vi "SubVI_ShifterControl.vi"(2 "Joystick Button":bool, 3 "Number of milliseconds\nto fire solenoids for":i32=200, 4 "Number of milliseconds to wait between shifts.\n~20ms precision.":i32=250) -> (0 "Low Gear Solenoid":bool=TRUE, 1 "High Gear Solenoid":bool=TRUE)   [LabVIEW 2017]
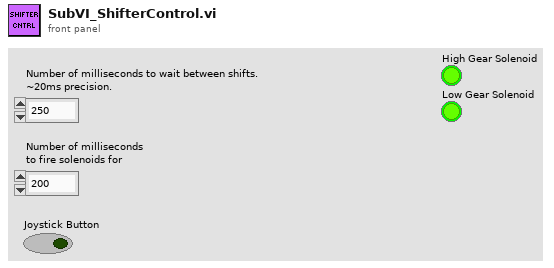
[diagram p1: front panel]
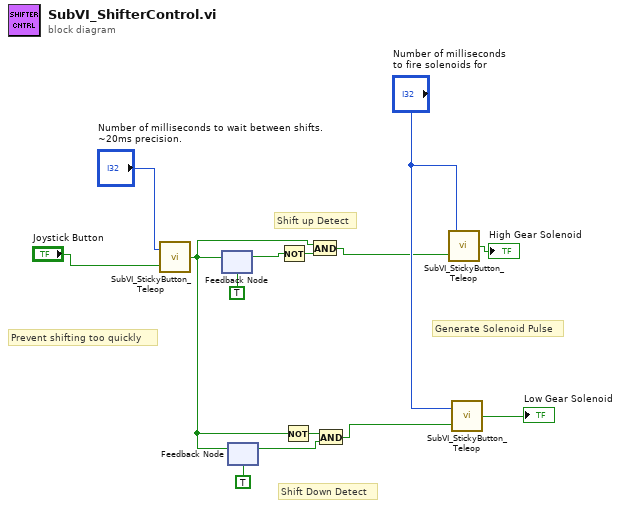
[diagram p0: block diagram]
diagram:
  # "Prevent shifting too quickly"
  # "Generate Solenoid Pulse"
  # "Shift Down Detect"
  # "Shift up Detect"
  n1 = call "SubVI_StickyButton_Teleop.vi"("Speedy Input"="Joystick Button", "Number of milliseconds to wait.\n~20ms precision."="Number of milliseconds to wait between shifts.\n~20ms precision.") -> ("Sticky Output"=w1:bool)
  n2 = feedback-in #1(w1) -> ()
  n3 = feedback #1(TRUE) -> (w7:bool)
  n4 = feedback-in #2(w1) -> ()
  n5 = feedback #2(TRUE) -> (w4:bool)
  n6 = Not(x=w7) -> (.not. x?=w9:bool)
  n7 = Not(x=w1) -> (.not. x?=w6:bool)
  n8 = And(x=w1, y=w9) -> (x .and. y?=w3:bool)
  n9 = And(x=w6, y=w4) -> (x .and. y?=w2:bool)
  n10 = call "SubVI_StickyButton_Teleop.vi"("Speedy Input"=w3, "Number of milliseconds to wait.\n~20ms precision."="Number of milliseconds\nto fire solenoids for") -> ("Sticky Output"=→"High Gear Solenoid":bool)
  n11 = call "SubVI_StickyButton_Teleop.vi"("Speedy Input"=w2, "Number of milliseconds to wait.\n~20ms precision."="Number of milliseconds\nto fire solenoids for") -> ("Sticky Output"=→"Low Gear Solenoid":bool)
